vi "Get Virtual Ports.vi"(8 "error in (no error)":errorcluster) -> (0 "error out":errorcluster, 3 "Serial Ports out":string[](array[string]))   [LabVIEW 2023, in "Listener.lvclass"]
uses:
  Listener.lvclass
  <vilib>/Utility/error.llb/whitespace.ctl
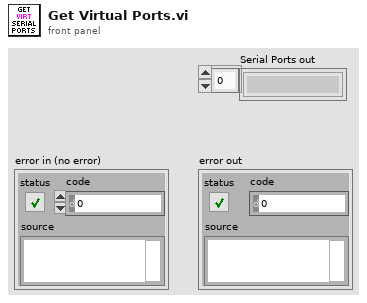
[diagram p1: front panel]
types:
  T1 = typedef "whitespace.ctl" = u16
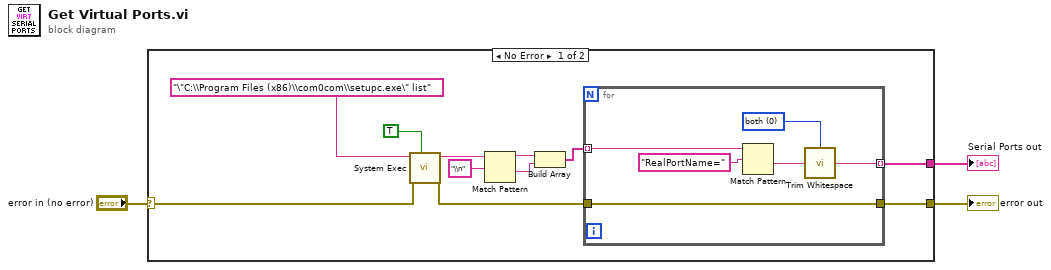
[diagram p0: block diagram]
diagram:
  n1 = case shown="No Error" "error in (no error)" {
    selector: "error in (no error)" -> [w5 w21]
    tunnel: [w7 w21] -> w3
    tunnel: [w6 _] -> w1
    frame No Error {
      n2 = call <vilib>:"System Exec.vi"("wait until completion? (T)"=TRUE, "error in (no error)"=w5, "command line"="\"C:\\Program Files (x86)\\com0com\\setupc.exe\" list") -> ("error out"=w4:errorcluster, "standard output"=w14:string)  [unwired: 5 in, 2 out]
      n3 = Match Pattern(string=w14, regular expression="\\n") -> (before substring=w13:string, after substring=w12:string)  [unwired: 1 in, 2 out]
      n4 = Build Array(w13, w12) -> (w8:string[])
      n5 = for {
        tunnel: w8 -> [w20] mode=indexing
        tunnel: w4 -> [w17]
        tunnel: [w17] -> w7
        tunnel: [w16] -> w6 mode=indexing
        w15 = T1 0 items=["both", "start of string", "end of string"] ("location (both)")
        n6 = Match Pattern(string=w20, regular expression="RealPortName=") -> (after substring=w18:string)  [unwired: 1 in, 3 out]
        n7 = call <vilib>:"Trim Whitespace.vi"("string"=w18, "location (both)"=w15) -> ("trimmed string"=w16:string)
      }
    }
    frame Error {
    }
  }
  "error out" <- w3
  "Serial Ports out" <- w1
